vi "multifit.vi"(6 "error in":errorcluster, 8 "List Peaks":string[][](table)=[["0", "2.298448", "56622.259938"], ["1", "3.693510", "568942.221745"], ["2", "3.986486", "85674.157303"], ["3", "12.564011", "20786.516854"]], 9 "List Parameter Fit In":dbl[][](array[numeric])=[[61895.26743495138, 2.295902819051137, 0.05132725028401794, 4549.770440475167, 604.272909684641, 0.00013211395312335064, 0.0005412786405150726, 657.5539740905274], [627372.2059878254, 3.692284511840813, 0.05677911685996556, 18601.27709030301, 3836.7824698281233, 8.354403497208279e-05, 0.0003643877607762332, 4160.712473210559], [74116.31578446296, 4.0147483591783155, 0.05085091795005294, 22427.950314927708, 307.3617647197942, 0.00014015981359792937, 0.0002809232075470725, 309.9731656877187], [28273.34836642687, 12.573977083982806, 0.10770256815937904, 51.48314892156685, 1352.5083475039019, 0.0004671472170224425, 0.004032939443201791, 1403.8484860391175]], 10 "List ROI In":dbl[][](array[numeric])=[[2.295902819051137, 0.12087567441886224, 747.0, 785.0, 2.233926550867361, 2.356038682169207, 6063.6329279938445, 123.14309366808929], [3.692284511840813, 0.1337148202052189, 1180.0, 1222.0, 3.625362152280503, 3.760328192140438, 67989.42495261344, 852.13028597231], [4.0147483591783155, 0.11975391177237468, 1283.0, 1320.0, 3.956350297651297, 4.075248951813621, 7193.497223633383, 69.57166423918198], [12.573977083982806, 0.2536395480153376, 3925.0, 4004.0, 12.446356900269128, 12.700221594291389, 5812.069028071378, 495.66499136986374]], 11 "Spectrum In":cluster{"Locations":dbl[], "Amplitudes":dbl[]}={"Locations"=array[8192 elements], "Amplitudes"=array[8192 elements]}) -> (1 "List Parameter Fit Out":dbl[][](array[numeric])=[[72985.42049784464, 2.29530433588858, 0.05722471236395812, -6719.954128683837, 3514.3279732857486, 7.641139969591555e-05, 0.0017646666004499732, 3559.3620345490303], [626906.4516896611, 3.6923878537448513, 0.056725550141628785, 19143.182126509742, 2756.558061175683, 9.742740047455971e-05, 0.00030585131086768315, 3020.7605065816324], [84952.09034117158, 4.0147539339226315, 0.05684400456146576, 11048.984691445543, 3382.5195465814695, 5.6421783276986587e-05, 0.0014333924536871097, 3422.1830799296517]], 2 "List ROI Out":dbl[][](array[numeric])=[[2.29530433588858, 0.13476419761712136, 745.0, 787.0, 2.2274995965883164, 2.3624656364482517, 7971.631104776367, 629.6678820155158], [3.6923878537448513, 0.1335886705835358, 1180.0, 1222.0, 3.625362152280503, 3.760328192140438, 67874.85518278569, 664.4170311995598], [4.0147539339226315, 0.13386763074225186, 1280.0, 1322.0, 3.9467098662327302, 4.0816759060926655, 9216.928010954993, 599.404820008226]], 3 "Spectrum Fitted":cluster{"Array":dbl[], "Array":dbl[]}, 4 "error out":errorcluster)   [LabVIEW 2023]
uses:
  control/List Fit peak.ctl
  <vilib>/Analysis/6fits.llb/Curve Fitting Criteria.ctl
  <vilib>/gmath/NumericalOptimization/Nonlinear Curve Fit LM bound.vi
  <vilib>/gmath/NI_Gmath.lvlib
  <vilib>/Analysis/NI_AALPro.lvlib
  queue/Front Panel Message Queue.lvlib
  <vilib>/gmath/NumericalOptimization/Nonlinear Curve Fit LM.vi
panel:
  in  "auto.X":bool
  in  "List reset":bool
  out "List Status":string[][](table)
  in  "List Fit Peak":T1[](array[typedef])
  in  "FWHM Bound Parameters (%)":dbl=60.0
  out "List MultiFit":dbl[][](array[numeric])
  out "R-square":dbl
  out "All FWHM":dbl[](array[numeric])
  out "All Parameters Fit":T2(array[cluster])
  in  "EnOffsetFit":bool
  in  "Erase":bool
  in  "mapping":enum16{"Y - Linear", "Y - Log"}(ring)
  in  "Fit":bool
  in  "Done":bool
  out "Spectrum":cluster{"Locations":dbl[], "Amplitudes":dbl[]}[](graph)
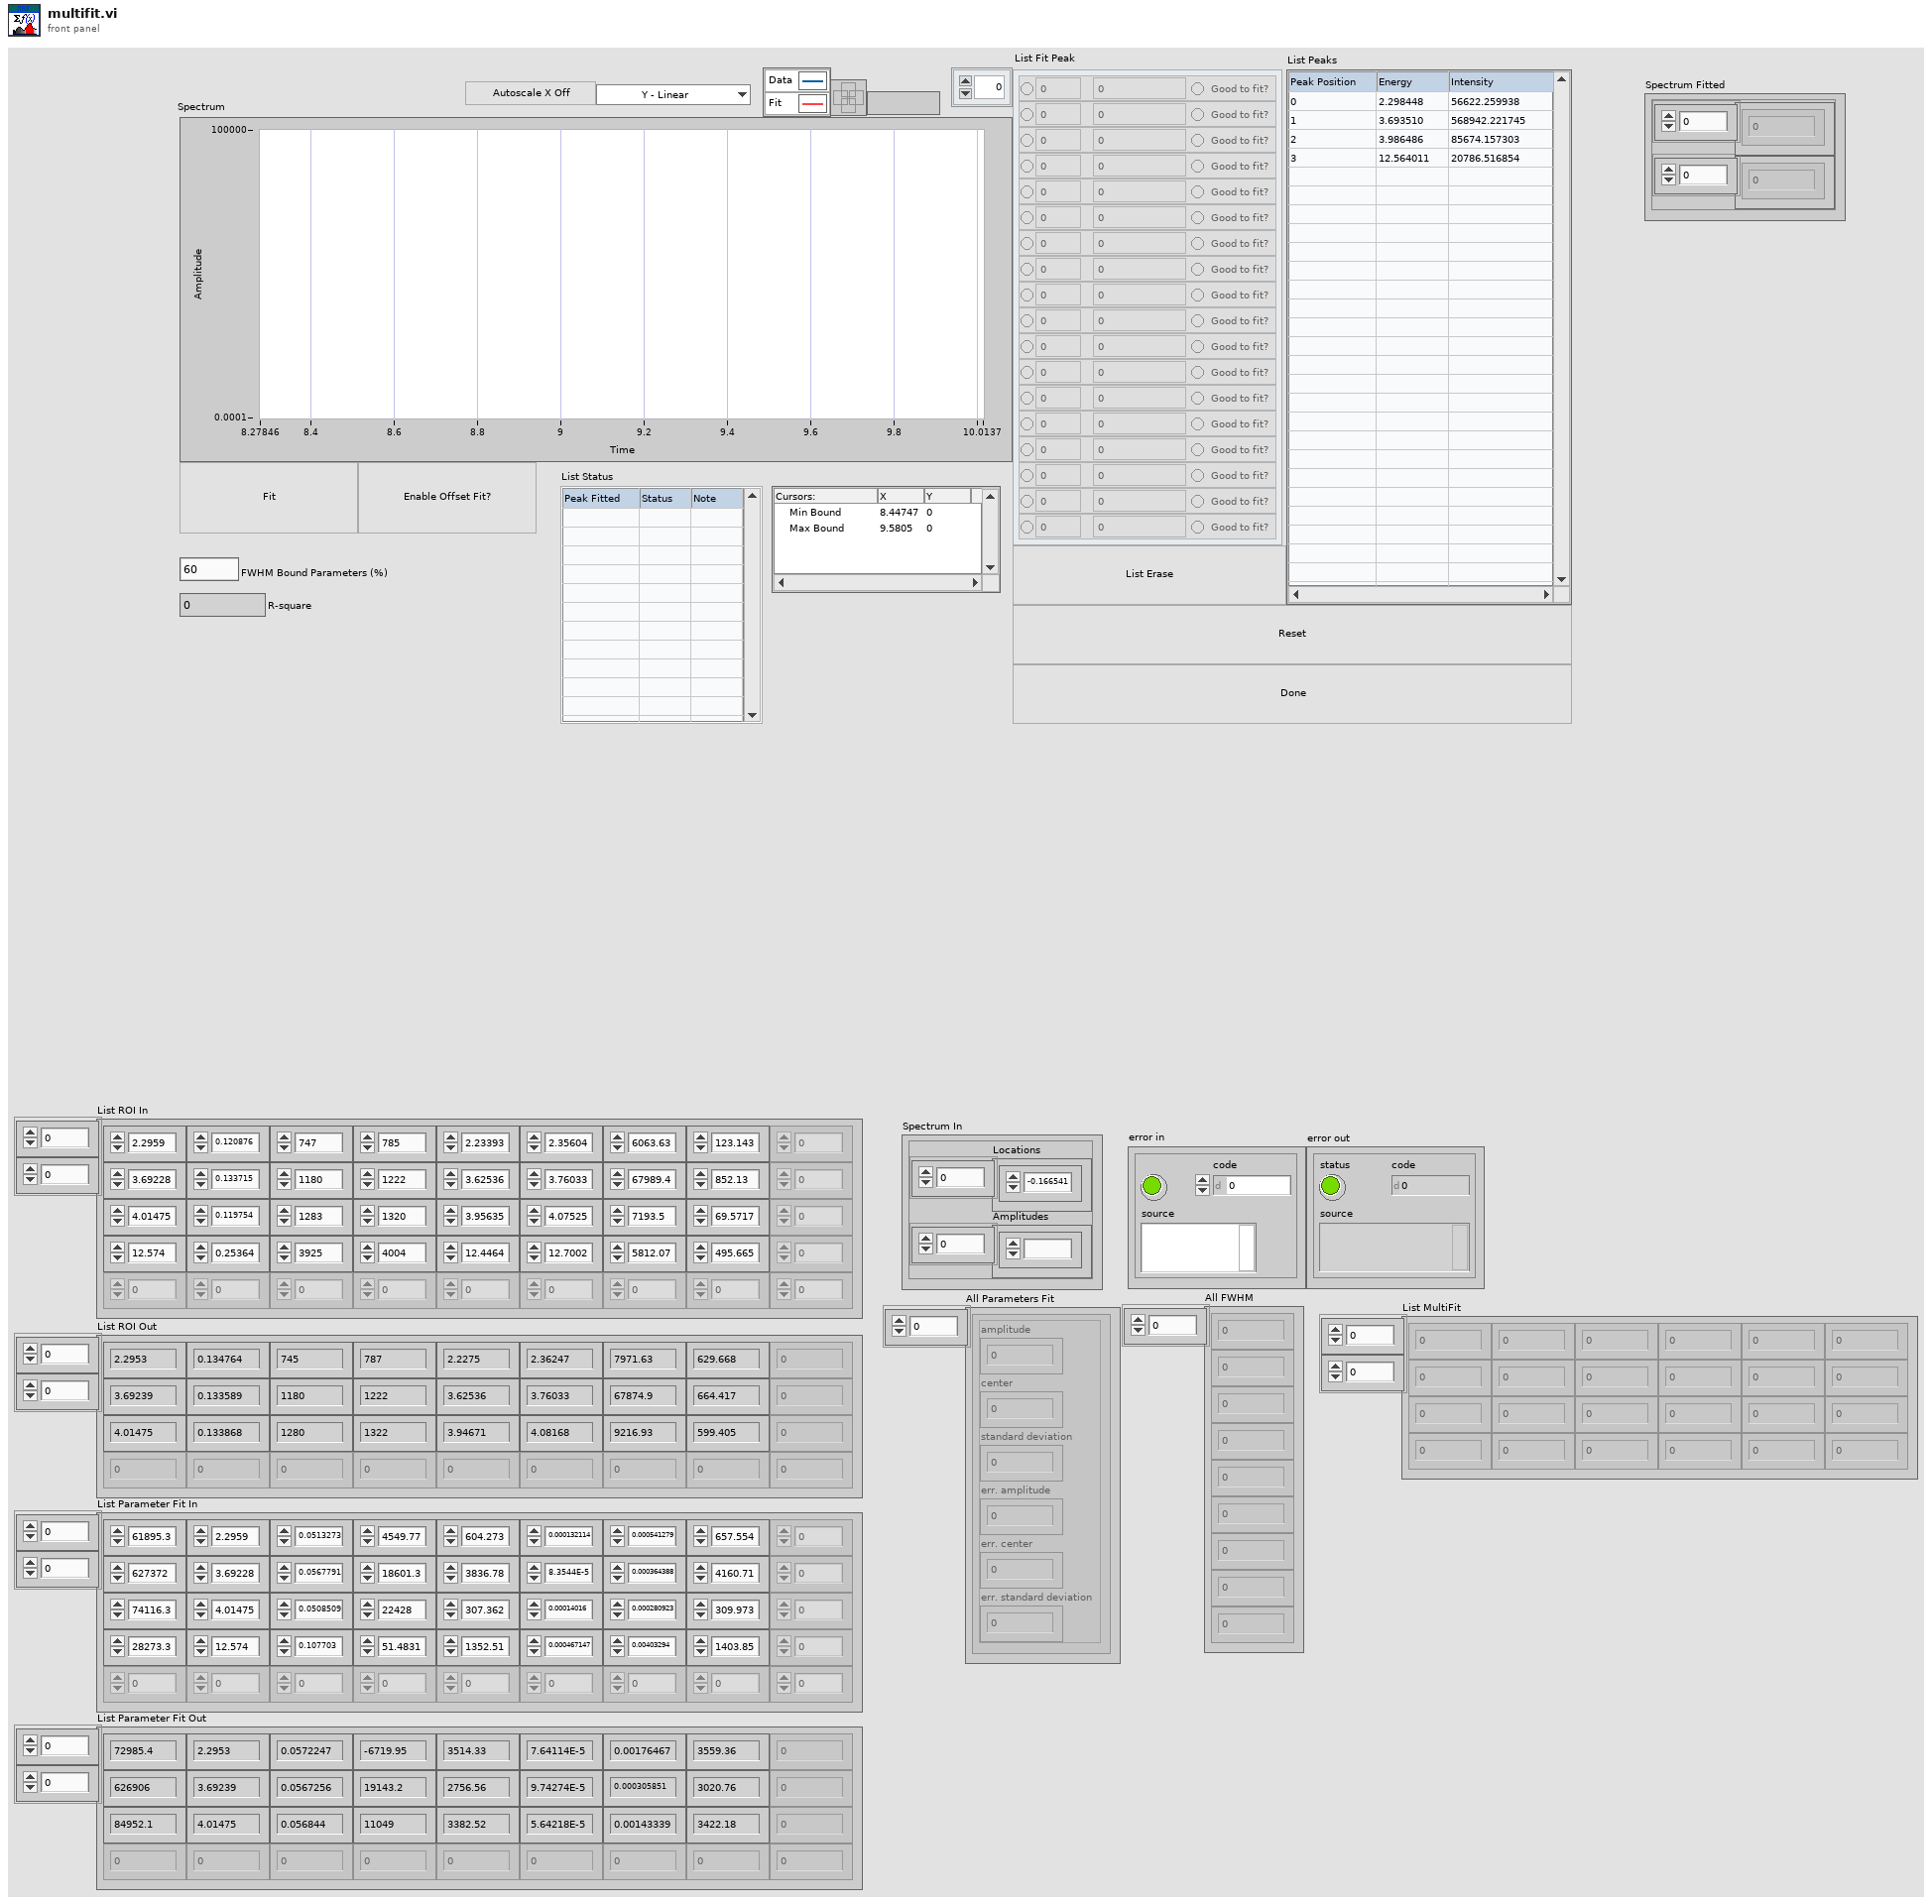
[diagram p1: front panel]
types:
  T1 = typedef "List Fit peak.ctl" = cluster{"Include":bool, "Position":dbl, "Energy":dbl, "good?":bool}
  T2 = cluster{"amplitude":dbl, "center":dbl, "standard deviation":dbl, "err. amplitude":dbl, "err. center":dbl, "err. standard deviation":dbl}[]
  T3 = typedef "Front Panel Message Queue.lvlib/load Message Queues.ctl" = cluster{"Main":refnum<queue>}
  T4 = cluster{"parameter minimum":dbl[], "parameter maximum":dbl[]}
  T5 = typedef "NI_AALPro.lvlib/Curve Fitting Criteria.ctl" = u16
  T6 = typedef "NI_Matrix.lvlib/RealMatrix.ctl" = dbl[][]
  T7 = cluster{"Array":dbl[], "best nonlinear fit":dbl[]}
  T8 = cluster{"Array":dbl[], "best nonlinear fit":dbl[]}[]
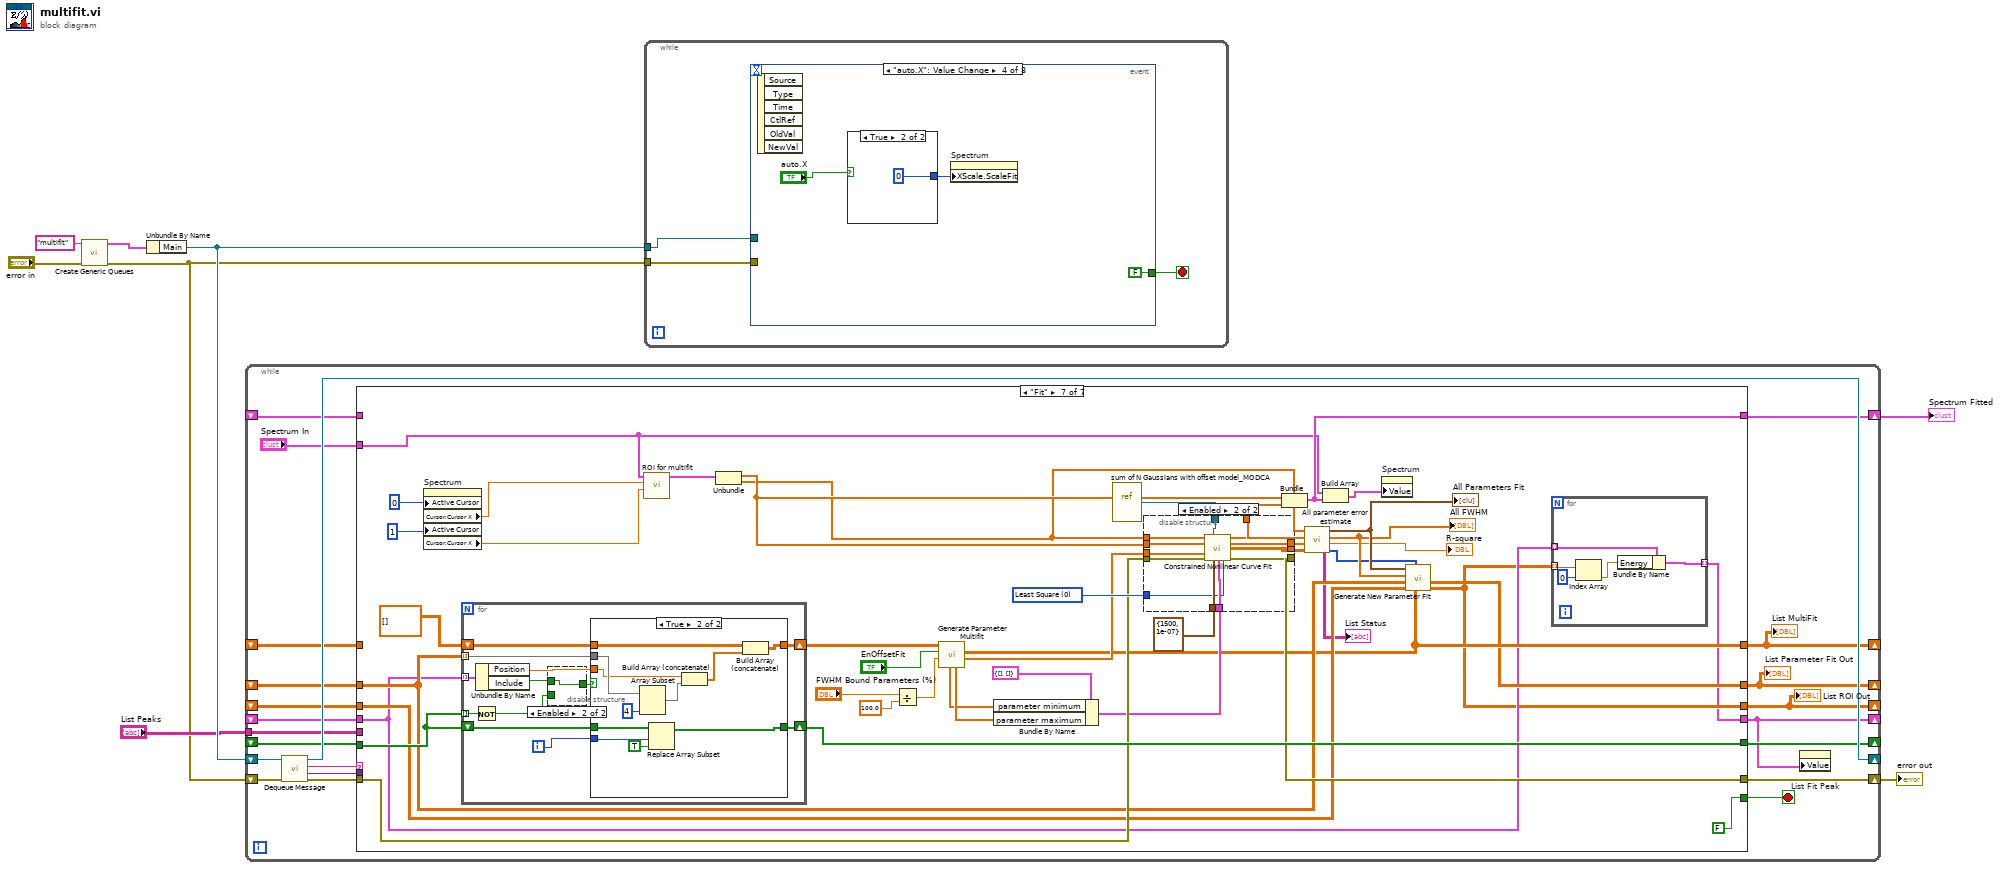
[diagram p0: block diagram]
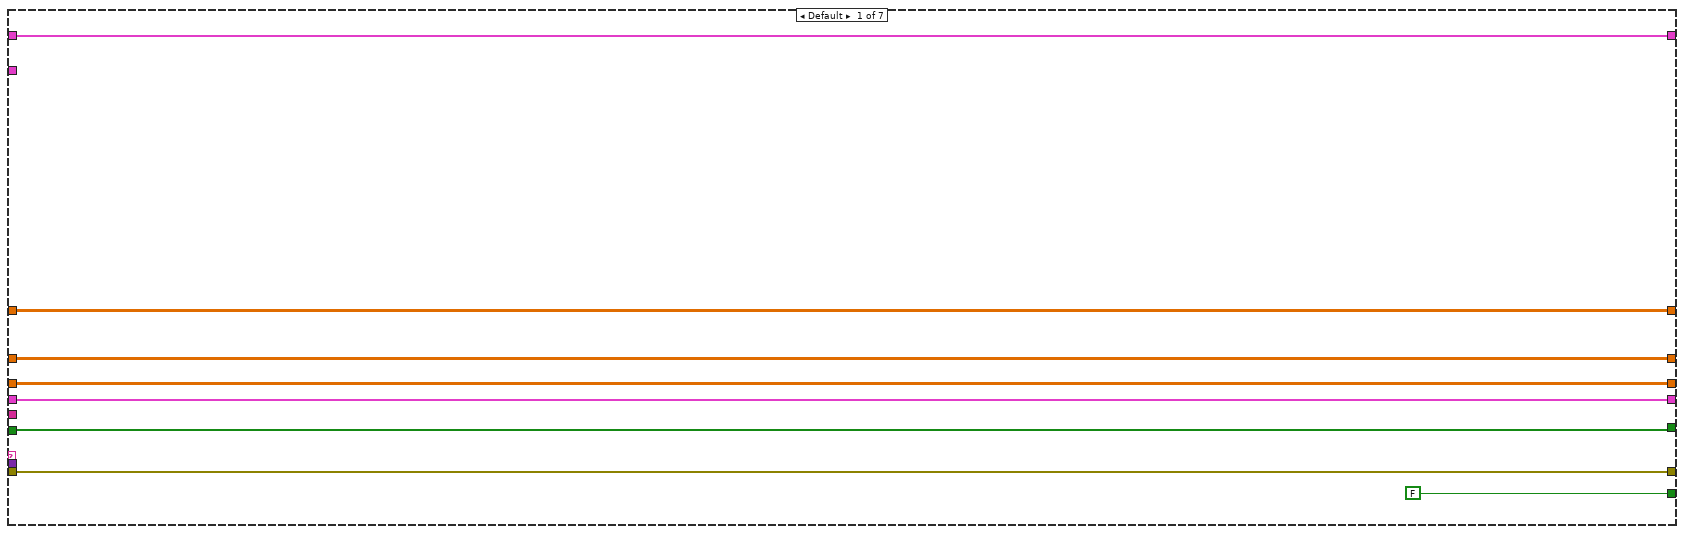
[diagram p2: hidden frame]
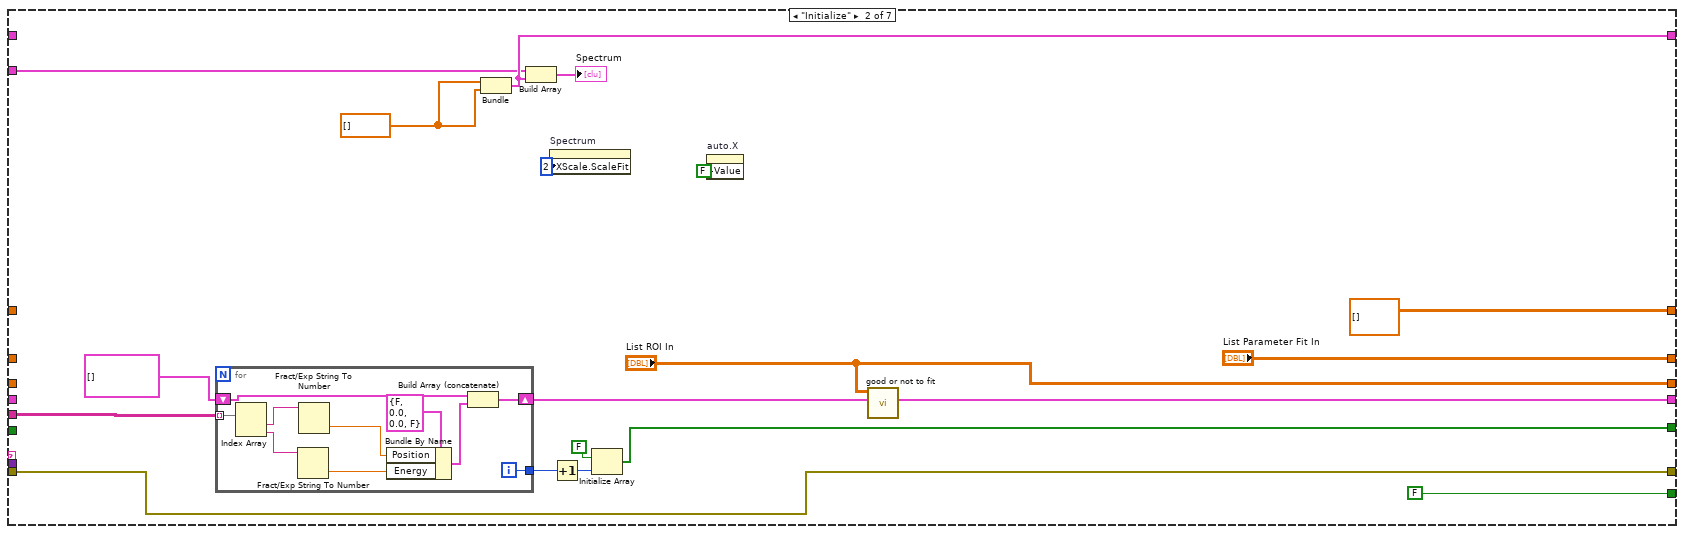
[diagram p3: hidden frame]
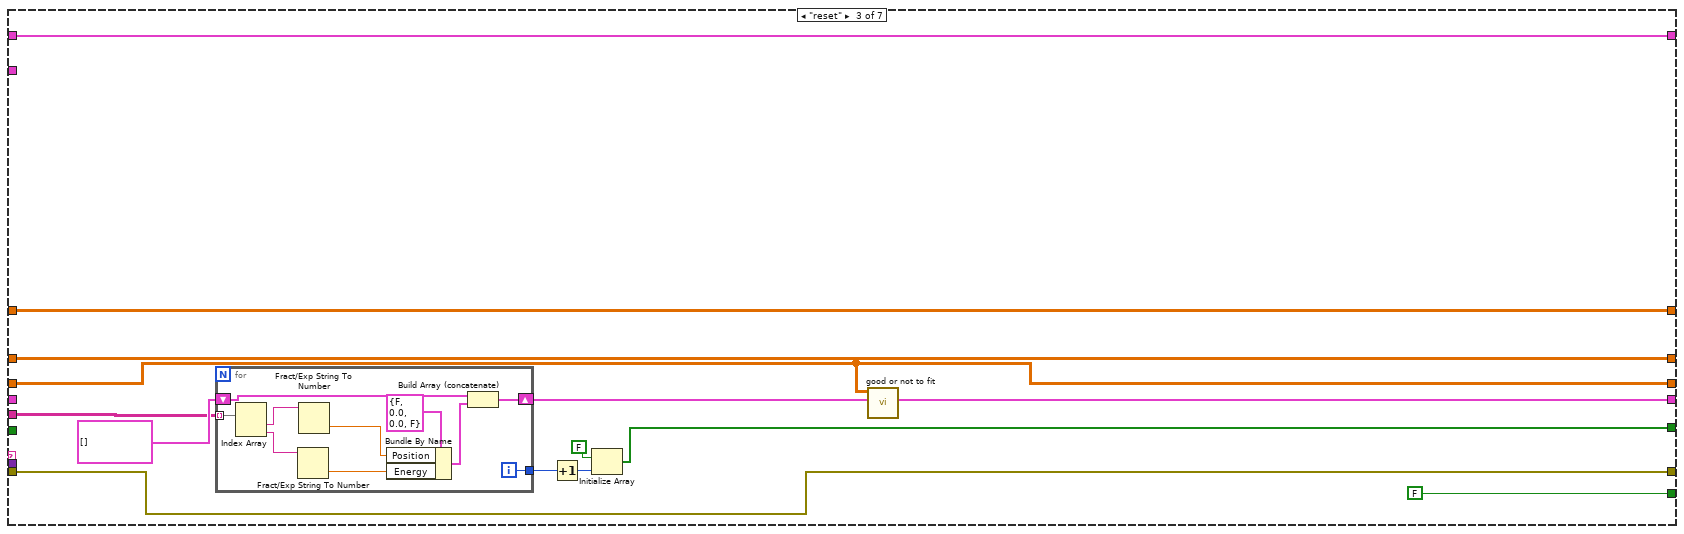
[diagram p4: hidden frame]
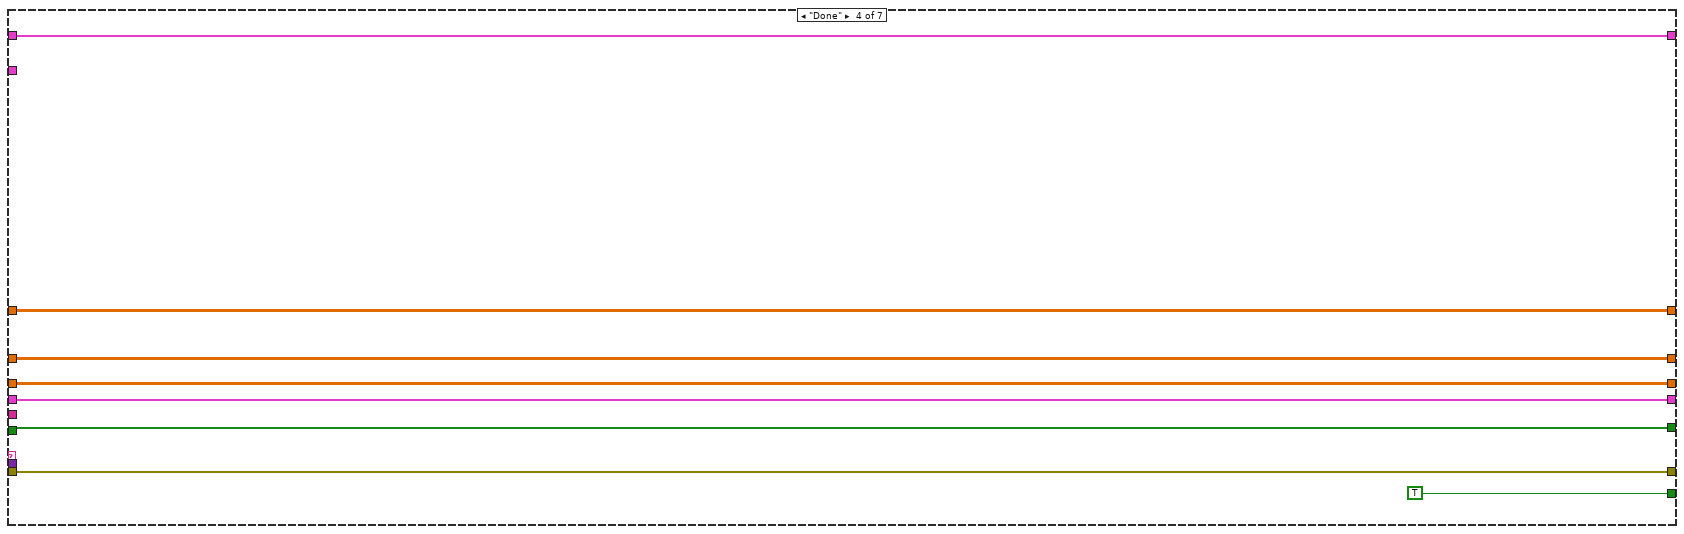
[diagram p5: hidden frame]
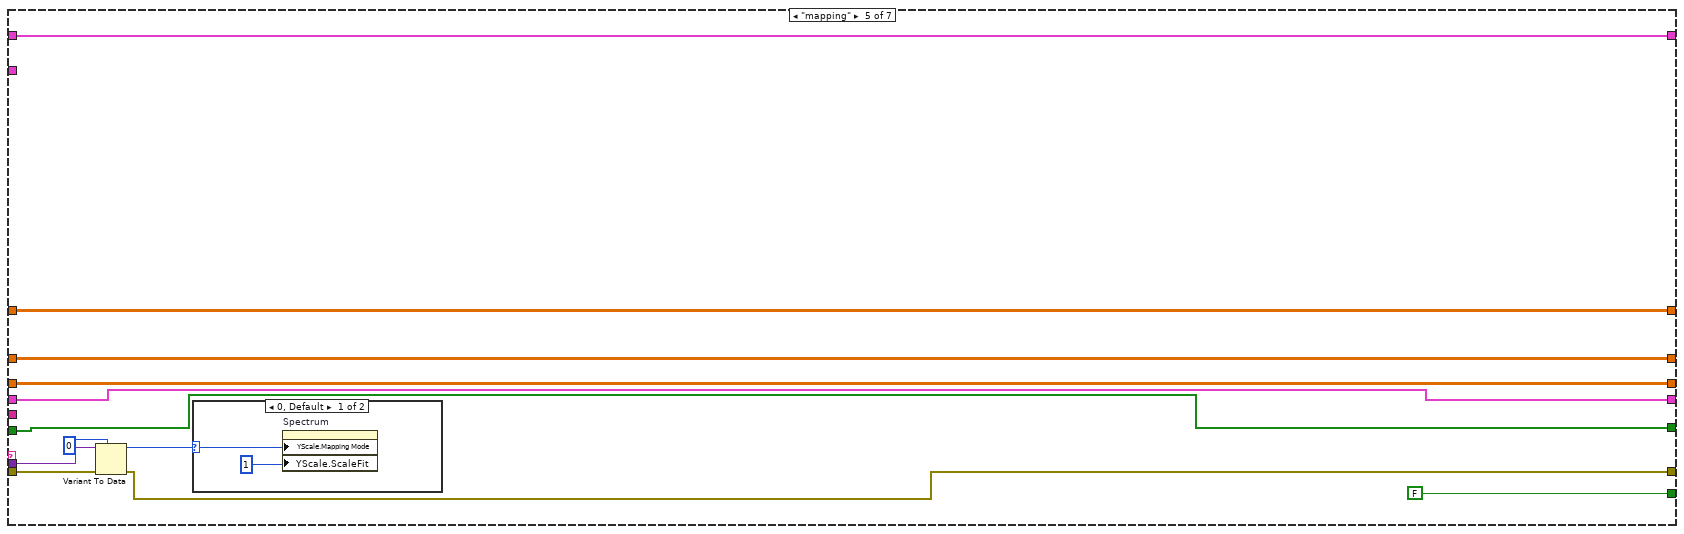
[diagram p6: hidden frame]
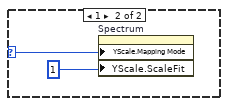
[diagram p7: hidden frame]
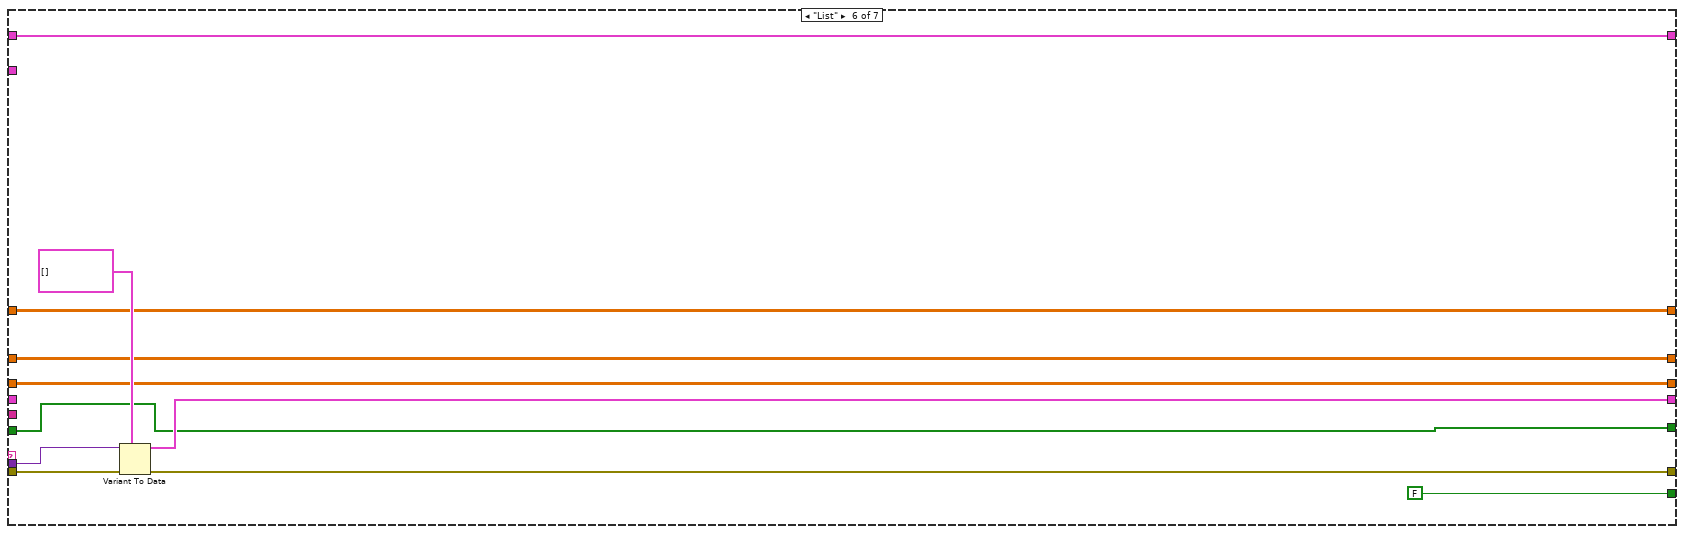
[diagram p8: hidden frame]
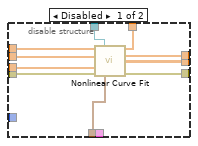
[diagram p9: hidden frame]
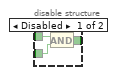
[diagram p10: hidden frame]
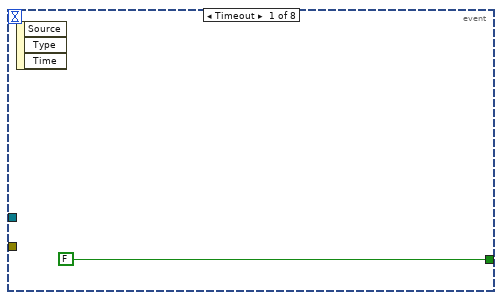
[diagram p12: hidden frame]
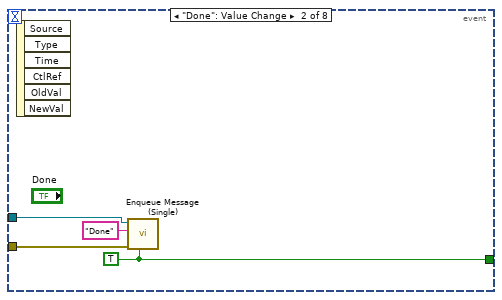
[diagram p13: hidden frame]
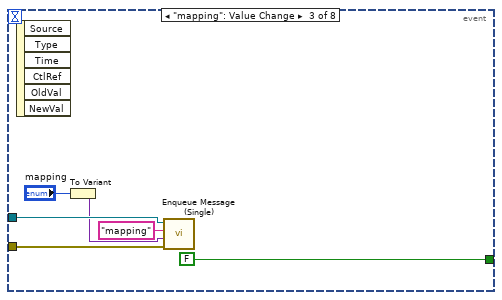
[diagram p14: hidden frame]
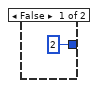
[diagram p15: hidden frame]
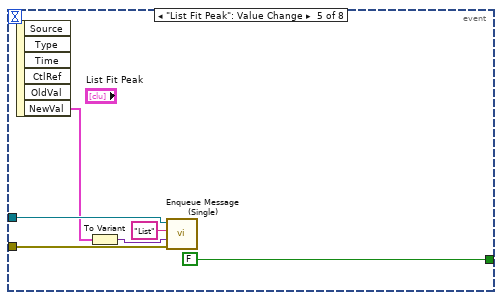
[diagram p16: hidden frame]
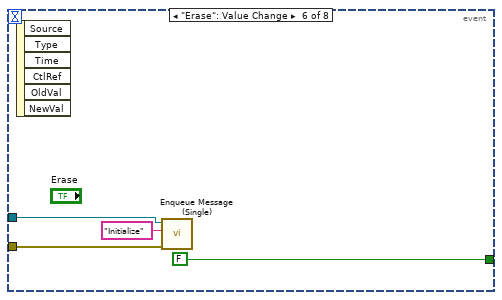
[diagram p17: hidden frame]
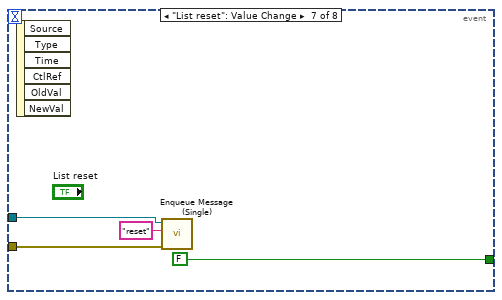
[diagram p18: hidden frame]
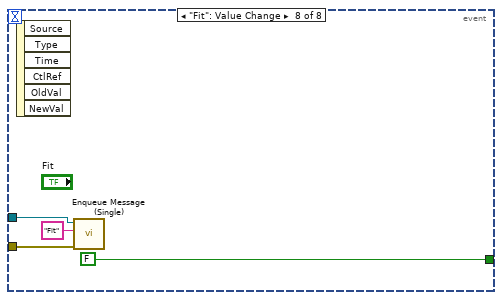
[diagram p19: hidden frame]
diagram:
  n1 = call "Create Generic Queues.vi"("error in (no error)"="error in", "name"="multifit") -> ("error out"=w1:errorcluster, "Message Queues"=w6:T3)  [unwired: 8 in]
  n2 = Unbundle By Name(w6) -> ("Main"=w5:refnum<queue>)
  n3 = while {
    shift-right: [w28] -> _
    shift-left: w5 -> [w30]
    shift-right: [w24] -> w2
    shift-left: w1 -> [w29]
    tunnel: "List Peaks" -> [w25]
    shift-right: [w9] -> _
    shift-left: _ -> [w23]
    shift-right: [w22] -> w3
    shift-left: _ -> [w21]
    shift-right: [w11] -> _
    shift-left: _ -> [w20]
    shift-right: [w13] -> _
    shift-left: _ -> [w19]
    shift-right: [w12] -> _
    shift-left: _ -> [w18]
    shift-right: [w17] -> _
    shift-left: _ -> [w16]
    stop <- w15 stop-if-true
    n4 = call "Dequeue Message.vi"("error in (no error)"=w29, "Message Queue"=w30) -> ("error out"=w27:errorcluster, "Message Data"=w14:variant, "Message"=w26:string, "dup Message Queue"=w28:refnum<queue>)  [unwired: 5 in, 1 out]
    n5 = case shown="\"Fit\"" w26 {
      tunnel: w27 -> [w38 w55 w79 w99 w111 w126 w152]
      tunnel: w25 -> [_ w56 w80 _ _ _ _]
      tunnel: [w37 w41 w72 w96 w101 w121 w127] -> w9
      tunnel: [w38 w55 w79 w99 w107 w123 w151] -> w24
      tunnel: w23 -> [w37 _ _ w96 w101 _ w129]
      tunnel: [w36 w53 w71 w92 w100 w116 w147] -> w22
      tunnel: w21 -> [w36 _ w71 w92 w100 w116 _]
      tunnel: [w35 dbl[][] [] ("List ROI In") w68 w93 w104 w117 w140] -> w11
      tunnel: w20 -> [w35 _ w68 w93 w104 w117 _]
      tunnel: [w34 "List Parameter Fit In" w69 w94 w103 w118 w139] -> w13
      tunnel: w19 -> [w34 _ w69 w94 w103 w118 w145]
      tunnel: [w33 "List ROI In" w70 w95 w102 w119 w128] -> w12
      tunnel: w18 -> [w33 _ w70 w95 w102 w119 w144]
      tunnel: [w32 w47 w75 w97 w105 w120 w168] -> w17
      tunnel: w16 -> [w32 _ _ w97 w105 w120 w170]
      tunnel: [FALSE FALSE FALSE TRUE FALSE FALSE FALSE] -> w15
      tunnel: w14 -> [_ _ _ _ w110 w125 _]
      tunnel: "Spectrum In" -> [_ w44 _ _ _ _ w130]
      frame Default {
      }
      frame "Initialize" {
        w54 = dbl[] []
        n6 = for {
          tunnel: w56 -> [w67] mode=indexing
          shift-right: [w64] -> w42
          shift-left: T1[] [] ("List Peak") -> [w66]
          tunnel: [w59] -> w48
          i -> [w59]
          n7 = Index Array(array=w67) -> (element #1=w63:string, element #2=w62:string)  [unwired: 2 in]
          n8 = Fract/Exp String To Number(string=w62) -> (number=w60:dbl)  [unwired: 3 in, 1 out]
          n9 = Fract/Exp String To Number(string=w63) -> (number=w61:dbl)  [unwired: 3 in, 1 out]
          n10 = Bundle By Name(cluster=T1 {"Include"=FALSE, "Position"=0.0, "Energy"=0.0, "good?"=FALSE} ("Fit Peak Cluster"), "Position"=w61, "Energy"=w60) -> (w65:T1)
          n11 = Build Array (concatenate)(w66, w65) -> (w64:T1[])
        }
        n12 = Bundle(w54, w54) -> (w53:cluster{dbl[], dbl[]})  [unwired: 1 in]
        n13 = Build Array(w44, w53) -> (→"Spectrum":cluster{"Locations":dbl[], "Amplitudes":dbl[]}[])
        n14 = property on="Spectrum" class="XYGraph (strict)"("XScale.ScaleFit"=u8 2 ("X Scale.Scale Fit")) -> ()  [unwired: 2 in, 2 out]
        n15 = Increment(x=w48) -> (x+1=w49:i32)
        n16 = Initialize Array(FALSE, w49) -> (w47:bool[])
        n17 = property on="auto.X" class="Bool (strict)"("Value"=FALSE ("auto.X")) -> ()  [unwired: 2 in, 2 out]
        n18 = call "good or not to fit.vi"("List Fit Peak In"=w42, "List ROI In"="List ROI In") -> ("List Fit Peak Out"=w41:T1[])  [unwired: 9 in]
      }
      frame "reset" {
        n19 = for {
          tunnel: w80 -> [w91] mode=indexing
          shift-right: [w88] -> w73
          shift-left: T1[] [] ("List Peak") -> [w90]
          tunnel: [w83] -> w76
          i -> [w83]
          n20 = Index Array(array=w91) -> (element #1=w87:string, element #2=w86:string)  [unwired: 2 in]
          n21 = Fract/Exp String To Number(string=w86) -> (number=w84:dbl)  [unwired: 3 in, 1 out]
          n22 = Fract/Exp String To Number(string=w87) -> (number=w85:dbl)  [unwired: 3 in, 1 out]
          n23 = Bundle By Name(cluster=T1 {"Include"=FALSE, "Position"=0.0, "Energy"=0.0, "good?"=FALSE} ("Fit Peak Cluster"), "Position"=w85, "Energy"=w84) -> (w89:T1)
          n24 = Build Array (concatenate)(w90, w89) -> (w88:T1[])
        }
        n25 = Increment(x=w76) -> (x+1=w77:i32)
        n26 = Initialize Array(FALSE, w77) -> (w75:bool[])
        n27 = call "good or not to fit.vi"("List Fit Peak In"=w73, "List ROI In"=w70) -> ("List Fit Peak Out"=w72:T1[])  [unwired: 9 in]
      }
      frame "Done" {
      }
      frame "mapping" {
        n28 = Variant To Data(error in=w111, type=u16 0, Variant=w110) -> (data=w108:u16, error out=w107:errorcluster)
        n29 = case shown="0, Default" w108 {
          selector: w108 -> [w113 w115]
          frame 0, Default {
            n30 = property on="Spectrum" class="XYGraph (strict)"("YScale.Mapping Mode"=w113, "YScale.ScaleFit"=u8 1 ("Y Scale.Scale Fit")) -> ()  [unwired: 2 in, 2 out]
          }
          frame 1 {
            n31 = property on="Spectrum" class="XYGraph (strict)"("YScale.Mapping Mode"=w115, "YScale.ScaleFit"=u8 1 ("Y Scale.Scale Fit")) -> ()  [unwired: 2 in, 2 out]
          }
        }
      }
      frame "List" {
        n32 = Variant To Data(error in=w126, type=T1[] [] ("NewVal"), Variant=w125) -> (data=w121:T1[], error out=w123:errorcluster)
      }
      frame "Fit" {
        w158 = T5 0 items=["Least Square", "Least Absolute Residual", "Bisquare"] ("method")
        n33 = property on="Spectrum" class="XYGraph (strict)"("Active Cursor"=u32 0, "Active Cursor"=u32 1) -> ("Cursor.Cursor X"=w133:dbl, "Cursor.Cursor X"=w132:dbl)  [unwired: 2 in, 2 out]
        n34 = for {
          tunnel: w145 -> [w206] mode=indexing
          tunnel: w129 -> [w209] mode=indexing
          shift-right: [w208] -> w161
          shift-left: dbl[][] [] ("Rearranged Parameter Fit") -> [w207]
          tunnel: w170 -> [w205] mode=indexing
          shift-right: [w199] -> w168
          shift-left: w170 -> [w201]
          i -> [w200]
          n35 = Not(x=w205) -> (.not. x?=w202:bool)
          n36 = Unbundle By Name(w209) -> ("Position"=w198:dbl, "Include"=w203:bool)
          n37 = disable-structure shown="Enabled" {
            disable-tunnel: [w212 w213] -> w204
            disable-tunnel: w203 -> [w211 w213]
            disable-tunnel: w202 -> [w210 _]
            frame Disabled {
              n38 = And(x=w211, y=w210) -> (x .and. y?=w212:bool)
            }
            frame Enabled {
            }
          }
          n39 = case shown="True" w204 {
            tunnel: [w215 w226] -> w208
            tunnel: w207 -> [w215 w225]
            tunnel: w206 -> [_ w220]
            tunnel: w201 -> [w214 w224]
            tunnel: w200 -> [_ w219]
            tunnel: [w214 w222] -> w199
            tunnel: w198 -> [_ w217]
            frame False {
            }
            frame True {
              n40 = Array Subset(array=w220, length=4) -> (w218:dbl[])  [unwired: 1 in]
              n41 = Replace Array Subset(array=w224, new element=TRUE ("new element/subarray"), index=w219) -> (w222:bool[])
              n42 = Build Array (concatenate)(w217, w218) -> (w216:dbl[])
              n43 = Build Array (concatenate)(w225, w216) -> (w226:dbl[][])
            }
          }
        }
        n44 = call "ROI for multifit.vi"("Cursor En Max"=w132, "Cursor En Min"=w133, "Spectrum In"=w130) -> ("Spectrum Reuced"=w131:cluster{"Array":dbl[], "Array":dbl[]})  [unwired: 8 in]
        n45 = Unbundle(w131) -> ("Array"=w149:dbl[], "Array"=w148:dbl[])
        n46 = Divide(x="FWHM Bound Parameters (%)", y=100.0) -> (x/y=w167:dbl)
        n47 = call "Generate Parameter Multifit.vi"("FWHM Bound Parameters (%)"=w167, "EnOffsetFit"="EnOffsetFit", "All Parameter Fit"=w161) -> ("Initial Conditions"=w150:dbl[], "Rearranged Parameter Fit"=w140:dbl[][], "Max Bound Condition"=w165:dbl[], "Min Bound Condition"=w164:dbl[])  [unwired: 4 in, 1 out]
        n48 = Bundle By Name(cluster=T4 {"parameter minimum"=[], "parameter maximum"=[]} ("parameter bounds"), "parameter minimum"=w164, "parameter maximum"=w165) -> (w146:T4)
        n49 = vi-ref "sum of N Gaussians with offset model_MODCA.vi"() -> (w153:refnum<vi>)
        n50 = disable-structure shown="Enabled" {
          disable-tunnel: w152 -> [w185 w196]
          disable-tunnel: [w184 w195] -> w151
          disable-tunnel: w153 -> [w183 w192]
          disable-tunnel: w149 -> [w182 w193]
          disable-tunnel: [w181 w190] -> w154
          disable-tunnel: [w180 w188] -> w155
          disable-tunnel: [w179 w189] -> w156
          disable-tunnel: w148 -> [w178 w194]
          disable-tunnel: w150 -> [w177 w191]
          disable-tunnel: cluster{"max iteration":i32, "tolerance":dbl} {"max iteration"=1500, "tolerance"=1e-07} ("termination") -> [w176 w197]
          disable-tunnel: w146 -> [_ w187]
          disable-tunnel: w158 -> [_ w186]
          frame Disabled {
            n51 = call-poly <vilib>:"Nonlinear Curve Fit.vi"("Y"=w178, "f(x,a)"=w183, "X"=w182, "initial parameters"=w177, "error in (no error)"=w185, "termination"=w176) -> ("best nonlinear fit"=w179:dbl[], "best fit parameters"=w180:dbl[], "covariance"=w181:T6, "error out"=w184:errorcluster)  [unwired: 4 in, 2 out]
          }
          frame Enabled {
            n52 = call-poly <vilib>:"Constrained Nonlinear Curve Fit.vi"("Y"=w194, "f(x,a)"=w192, "X"=w193, "initial parameters"=w191, "error in (no error)"=w196, "termination"=w197, "parameter bounds"=w187, "method"=w186) -> ("best nonlinear fit"=w189:dbl[], "best fit parameters"=w188:dbl[], "covariance"=w190:T6, "error out"=w195:errorcluster)  [unwired: 2 in, 2 out]
          }
        }
        n53 = Bundle("Array"=w149, "best nonlinear fit"=w156) -> (w147:T7)  [unwired: 1 in]
        n54 = call "All parameter error estimate.vi"("covariance"=w154, "best fit parameters"=w155, "best nonlinear fit"=w156, "Y"=w148) -> ("Status"=w137:i32[], "R-square"=→"R-square":dbl, "All FWHM"=w142:dbl[], "All Parameters Fit"=w143:T2, "List Status"=→"List Status":string[][])  [unwired: 3 in]
        "All Parameters Fit" <- w143
        "All FWHM" <- w142
        n55 = Build Array(w130, w147) -> (w159:T8)
        n56 = property on="Spectrum" class="XYGraph (strict)"("Value"=w159) -> ()  [unwired: 2 in, 2 out]
        n57 = call "Generate New Parameter Fit.vi"("Rearranged Parameter Fit"=w140, "Status"=w137, "List ROI In"=w144, "List MultiFit In"=w145, "All FWHM"=w142, "All Parameters Fit"=w143) -> ("List ROI Out"=w128:dbl[][], "List MultiFit Out"=w139:dbl[][])  [unwired: 4 in]
        n58 = for {
          tunnel: w129 -> [w175] mode=indexing
          tunnel: w128 -> [w173] mode=indexing
          tunnel: [w171] -> w127 mode=indexing
          n59 = Index Array(array=w173, index=0) -> (element=w174:dbl)
          n60 = Bundle By Name(cluster=w175, "Energy"=w174) -> (w171:T1)
        }
      }
    }
    "List Parameter Fit Out" <- w13
    "List ROI Out" <- w12
    "List MultiFit" <- w11
    n61 = property on="List Fit Peak" class="Arr (strict)"("Value"=w9) -> ()  [unwired: 2 in, 2 out]
  }
  "error out" <- w2
  "Spectrum Fitted" <- w3
  n62 = while {
    tunnel: w5 -> [w228]
    tunnel: w1 -> [w227]
    stop <- w229 stop-if-true
    n63 = event shown="[3] \"auto.X\": Value Change" {
      selector: _ -> [_ _ _ _ _ _ _ _]
      dyn-events: _ -> [_ _ _ _ _ _ _ _]
      timeout: _ -> [_ _ _ _ _ _ _ _]
      tunnel: [FALSE w231 FALSE FALSE ("Priority Message? (F)") FALSE FALSE FALSE FALSE] -> w229
      tunnel: w227 -> [_ w234 w237 _ w250 w253 w257 w260]
      tunnel: w228 -> [_ w233 w238 _ w249 w252 w256 w261]
      event Timeout {
        n64 = event-data() -> ()  [unwired: 1 in, 3 out]
      }
      event "Done": Value Change {
        w231 = TRUE ("Priority Message? (F)")
        n65 = event-data() -> ()  [unwired: 1 in, 6 out]
        n66 = call "Enqueue Message (Single).vi"("Priority Message? (F)"=w231, "error in (no error)"=w234, "Message"="Done", "Message Queue"=w233) -> ()  [unwired: 6 in, 2 out]
      }
      event "mapping": Value Change {
        n67 = event-data() -> ()  [unwired: 1 in, 6 out]
        n68 = To Variant(anything="mapping") -> (Variant=w235:variant)
        n69 = call "Enqueue Message (Single).vi"("error in (no error)"=w237, "Message Data"=w235, "Message"="mapping", "Message Queue"=w238) -> ()  [unwired: 6 in, 2 out]
      }
      event "auto.X": Value Change {
        n70 = event-data() -> ()  [unwired: 1 in, 6 out]
        n71 = case shown="True" "auto.X" {
          tunnel: [u8 2 ("X Scale.Scale Fit") u8 0 ("X Scale.Scale Fit")] -> w242
          frame False {
          }
          frame True {
          }
        }
        n72 = property on="Spectrum" class="XYGraph (strict)"("XScale.ScaleFit"=w242) -> ()  [unwired: 2 in, 2 out]
      }
      event "List Fit Peak": Value Change {
        n73 = event-data() -> ("NewVal"=w246:T1[])  [unwired: 1 in, 5 out]
        n74 = To Variant(anything=w246) -> (Variant=w247:variant)
        n75 = call "Enqueue Message (Single).vi"("error in (no error)"=w250, "Message Data"=w247, "Message"="List", "Message Queue"=w249) -> ()  [unwired: 6 in, 2 out]
      }
      event "Erase": Value Change {
        n76 = event-data() -> ()  [unwired: 1 in, 6 out]
        n77 = call "Enqueue Message (Single).vi"("error in (no error)"=w253, "Message"="Initialize", "Message Queue"=w252) -> ()  [unwired: 7 in, 2 out]
      }
      event "List reset": Value Change {
        n78 = event-data() -> ()  [unwired: 1 in, 6 out]
        n79 = call "Enqueue Message (Single).vi"("error in (no error)"=w257, "Message"="reset", "Message Queue"=w256) -> ()  [unwired: 7 in, 2 out]
      }
      event "Fit": Value Change {
        n80 = event-data() -> ()  [unwired: 1 in, 6 out]
        n81 = call "Enqueue Message (Single).vi"("error in (no error)"=w260, "Message"="Fit", "Message Queue"=w261) -> ()  [unwired: 7 in, 2 out]
      }
    }
  }
